vi "Grid.vi"() -> ()   [LabVIEW 2017]
panel:
  in  "Segment":i32=25
  in  "Grid sizes":i32(ring)=2 items=["2*2"=2, "3*3"=3, "4*4"=4]
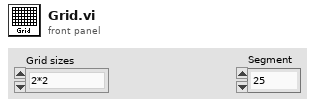
[diagram p1: front panel]
types:
  T1 = enum16{"Full", "Half", "Quarter", "Eighth", "Sixteenth"}
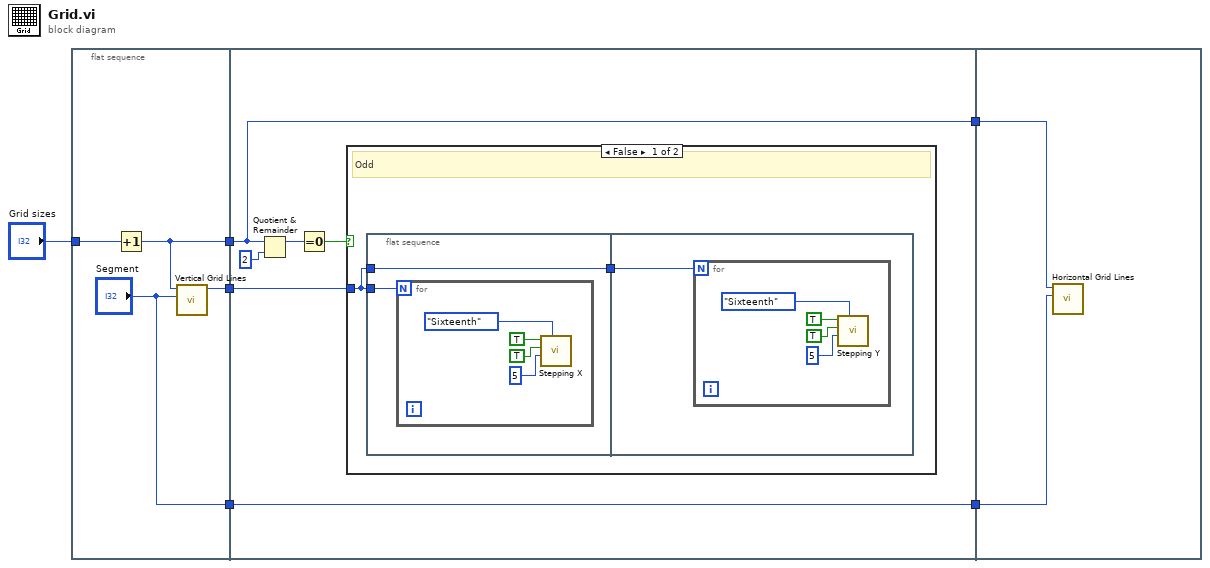
[diagram p0: block diagram]
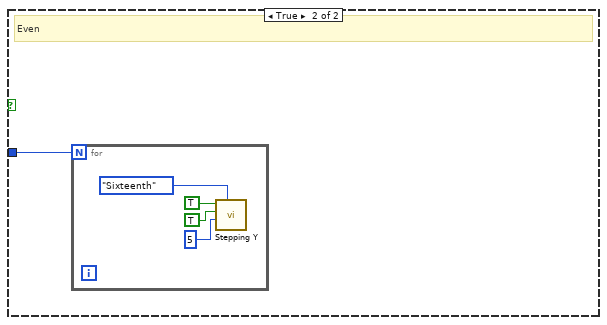
[diagram p2: hidden frame]
diagram:
  n1 = flat-sequence {
    tunnel: "Grid sizes" -> [w10]
    tunnel: [w9] -> w5
    tunnel: ["Segment"] -> w3
    tunnel: [w7] -> w1
    tunnel: w5 -> [w11]
    tunnel: [w11] -> w4
    tunnel: w3 -> [w12]
    tunnel: [w12] -> w2
    tunnel: w1 -> [w13]
    tunnel: w4 -> [w36]
    tunnel: w2 -> [w35]
    frame #0 {
      n2 = Increment(x=w10) -> (x+1=w9:i32)
      n3 = call "Vertical Grid Lines.vi"("Segment"="Segment", "No. of veritcal lines"=w9) -> ("Length"=w7:i32)  [unwired: 8 in, 1 out]
    }
    frame #1 {
      n4 = Quotient & Remainder(x=w11, y=2) -> (x-y*floor(x/y)=w16:i32)  [unwired: 1 out]
      n5 = Equal To 0?(x=w16) -> (x = 0?=w15:bool)
      n6 = case shown="False" w15 {
        tunnel: w13 -> [w17 w30]
        frame False {
          # "Odd"
          n7 = flat-sequence {
            tunnel: w17 -> [w20]
            tunnel: [w19] -> w18
            tunnel: w17 -> [w19]
            tunnel: w18 -> [w25]
            frame #0 {
              n8 = for {
                N: w20 -> [_]
                n9 = call "Stepping X.vi"("Microstep size"=T1."Sixteenth", "Speed"=u32 5, "Direction"=TRUE, "Enable"=TRUE) -> ()  [unwired: 7 in, 1 out]
              }
            }
            frame #1 {
              n10 = for {
                N: w25 -> [_]
                n11 = call "Stepping Y.vi"("Microstep size"=T1."Sixteenth", "Speed"=u32 5, "Direction"=TRUE, "Enable"=TRUE) -> ()  [unwired: 7 in, 1 out]
              }
            }
          }
        }
        frame True {
          # "Even"
          n12 = for {
            N: w30 -> [_]
            n13 = call "Stepping Y.vi"("Microstep size"=T1."Sixteenth", "Speed"=u32 5, "Direction"=TRUE, "Enable"=TRUE) -> ()  [unwired: 7 in, 1 out]
          }
        }
      }
    }
    frame #2 {
      n14 = call "Horizontal Grid Lines.vi"("Segment"=w35, "No. of horizontal lines"=w36) -> ()  [unwired: 9 in, 1 out]
    }
  }
